vi "free_pack.vi"(3 "error in":errorcluster, 5 "p":u64) -> (0 "error out":errorcluster)   [LabVIEW 2019, in "msgpack.lvlib"]
doc: "Closes the msgpack object and frees any memory associated with it. Do not use the pointer returned by get_packed_data after calling this VI"
uses:
  msgpack.lvlib
  msgpackalt.dll
panel:
  # "msgpack"
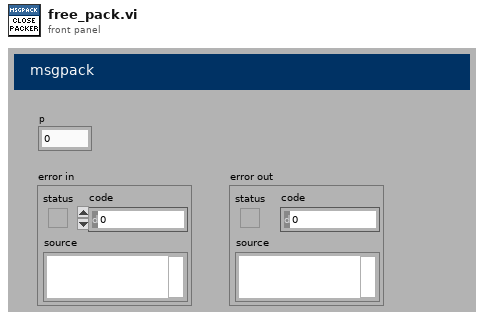
[diagram p1: front panel]
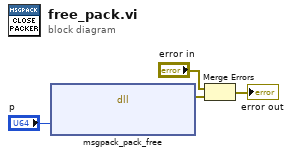
[diagram p0: block diagram]
diagram:
  n1 = dll-call lib="C:/Users/Patrick/Documents/GitHub/Instrument-Framework/lvsrc/SMOs/JSON-RPC-2019/lv-venv/lv.lib/vi.lib/addons/msgpack/msgpackalt.dll" fn="msgpack_pack_free"("p"="p") -> (error out=w3:errorcluster)  [unwired: 5 in, 1 out]
  n2 = Merge Errors("error in", w3) -> (→"error out":errorcluster)
